vi "select_stim.vi"(3 "n catch":u16, 4 "n stim":u16, 5 "catch array":u8[](array[numeric]), 6 "stim array":dbl[](array[numeric])) -> (0 "catch":bool, 1 "stim amp":dbl format="%.2f", 2 "stim idx":i32)   [LabVIEW 2015]
uses:
  <vilib>/Analysis/1siggen.llb/Riffle Array (DBL).vi
  <vilib>/Analysis/NI_AALBase.lvlib
panel:
  # "(see Block Diagram)"
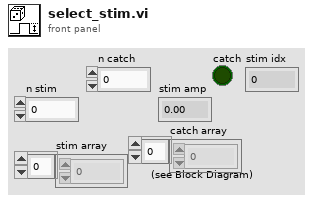
[diagram p1: front panel]
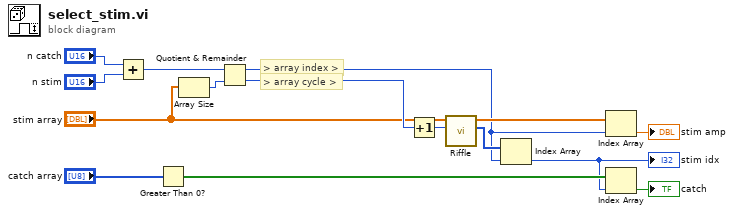
[diagram p0: block diagram]
diagram:
  # "> array index >"
  # "> array cycle >"
  n1 = Add(x="n catch", y="n stim") -> (x+y=w4:u16)
  n2 = Greater Than 0?(x="catch array") -> (x > 0?=w5:bool[])
  n3 = Array Size(array="stim array") -> (size(s)=w11:i32)
  n4 = Quotient & Remainder(x=w4, y=w11) -> (x-y*floor(x/y)=w8:i32, floor(x/y)=w15:i32)
  n5 = Increment(x=w15) -> (x+1=w14:i32)
  n6 = call-poly <vilib>:"Riffle.vi"("seed"=w14, "X"="stim array") -> ("Riffled Index"=w9:i32[], "Riffled {X}"=w10:dbl[])  [unwired: 7 in, 1 out]
  n7 = Index Array(array=w9, index=w8) -> (element=w1:i32)
  "stim idx" <- w1
  n8 = Index Array(array=w10, index=w8) -> (element=→"stim amp":dbl)
  n9 = Index Array(array=w5, index=w1) -> (element=→"catch":bool)
